vi "1. Vision Acquisition.vi"() -> ()   [LabVIEW 2019]
doc: "c 2020 ReMiSYS All rights reserved."
panel:
  in  "Stop (F)":bool
  out "Image Out":T1(plugin-control)
  # "Snapshot  (v)\nSnapshot Mode¡XDetermines if the control makes a copy of the image or has a reference to the image. When you enable the Snapshot Mode, \nif the inspection image changes later in your application, the Image Display control continues to display the image as it was when the image was wired into the Image Display control. \n\nEnabling the Snapshot Mode may reduce the speed of your application because the control makes a copy of the image. \nEnable this property when you want to display a snapshot of the image in time. \nDisable this property when you need to display results quickly, such as during a grab acquisition. The Snapshot Mode property is disabled by default.\n\nZoom to fit (v)\n\nPalette/Greyscale\nhttp://zone.ni.com/reference/en-XX/help/370281AG-01/imaqvision/imaq_getpalette/\n\nImage Display (Silver)\nhttps://knowledge.ni.com/KnowledgeArticleDetails?id=kA00Z000000P7klSAC&l=zh-TW"
  # "c 2022 ReMiSYS All rights reserved."
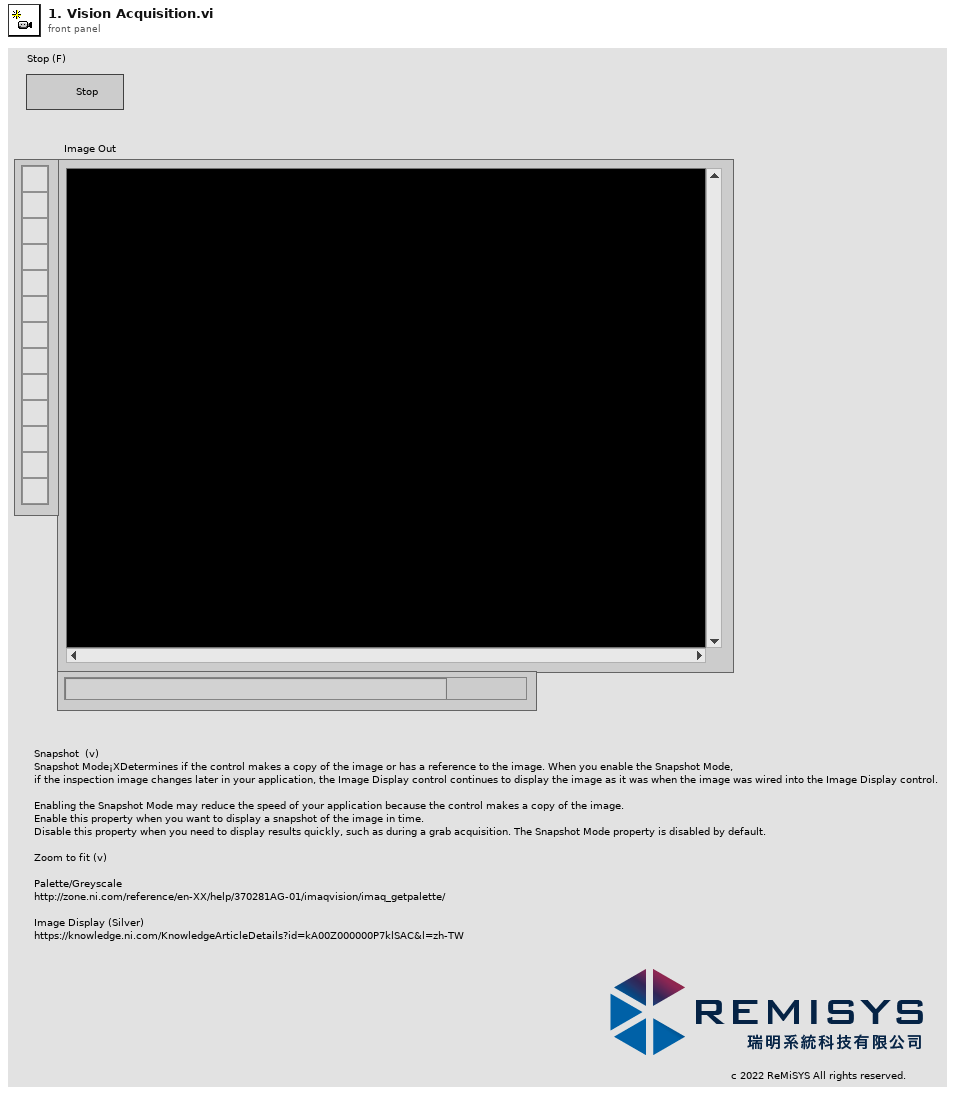
[diagram p1: front panel]
types:
  T1 = typedef "IMAQ Image.ctl" = refnum<image>
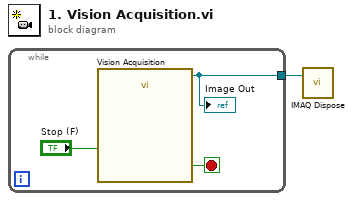
[diagram p0: block diagram]
diagram:
  n1 = while {
    tunnel: [w2] -> w1
    stop <- w3 stop-if-true
    n2 = call "Vision Acquisition"("Stop (F)"="Stop (F)") -> ("Image Out"=w2:T1, "Stopped"=w3:bool)  [unwired: 24 in, 1 out]
    "Image Out" <- w2
  }
  n3 = call "IMAQ Dispose"("Image"=w1) -> ()  [unwired: 5 in, 1 out]
